vi "Get Validation Information From Module Connections.vi"(8 "error in":errorcluster, 10 "module connection information":T2[](array[typedef])) -> (0 "error out":errorcluster, 2 "validation information":T1)   [LabVIEW 2019, in "Routing and Faulting Scripting.lvlib"]
uses:
  Routing and Faulting Scripting.lvlib
  Types/Module Information.ctl
  Shared/Routing and Faulting Hardware API/Types/Possible Connections for Endpoint.ctl
  Validation Information.ctl
  Shared/Routing and Faulting Hardware API/Routing and Faulting Hardware API.lvlib
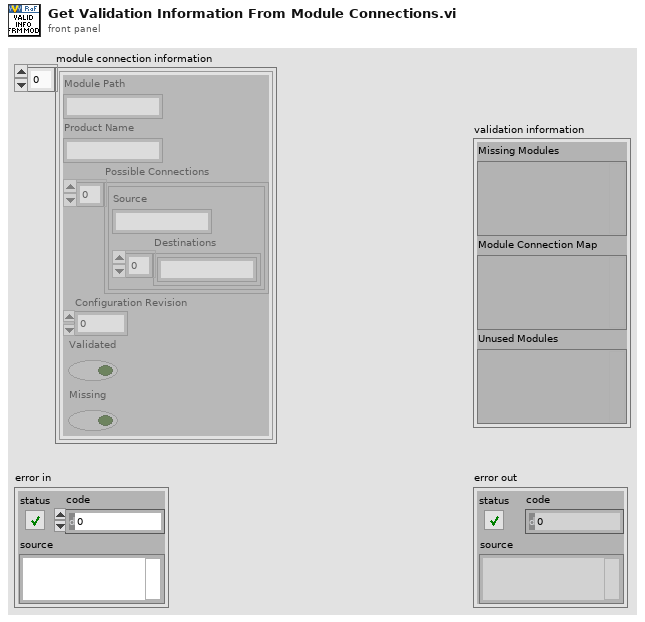
[diagram p1: front panel]
types:
  T1 = typedef "Routing and Faulting Scripting.lvlib/Validation Information.ctl" = cluster{"Missing Modules":variant, "Module Connection Map":variant, "Unused Modules":variant}
  T2 = typedef "Routing and Faulting Scripting.lvlib/Module Information.ctl" = cluster{"Module Path":string, "Product Name":string, "Possible Connections":T3[], "Configuration Revision":u32, "Validated":bool, "Missing":bool}
  T3 = typedef "Routing and Faulting Hardware API.lvlib/Possible Connections for Endpoint.ctl" = cluster{"Source":string, "Destinations":string[]}
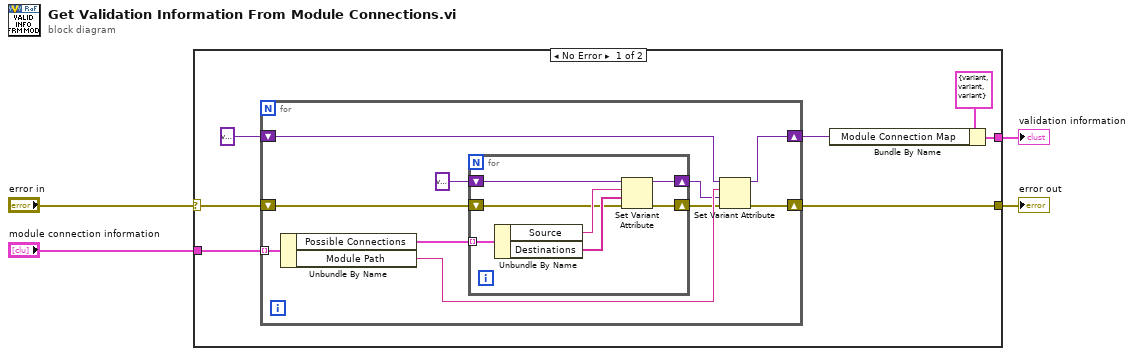
[diagram p0: block diagram]
diagram:
  n1 = case shown="No Error" "error in" {
    selector: "error in" -> [w5 w29]
    tunnel: "module connection information" -> [w8 _]
    tunnel: [w7 w29] -> w3
    tunnel: [w6 _] -> w2
    frame No Error {
      n2 = for {
        shift-right: [w12] -> w9
        shift-left: variant -> [w13]
        tunnel: w8 -> [w20] mode=indexing
        shift-right: [w14] -> w7
        shift-left: w5 -> [w16]
        n3 = Unbundle By Name(w20) -> ("Possible Connections"=w19:T3[], "Module Path"=w18:string)
        n4 = for {
          shift-right: [w24] -> w17
          shift-left: variant -> [w28]
          tunnel: w19 -> [w27] mode=indexing
          shift-right: [w22] -> w15
          shift-left: w16 -> [w23]
          n5 = Unbundle By Name(w27) -> ("Source"=w26:string, "Destinations"=w25:string[])
          n6 = Set Variant Attribute(Variant=w28, name=w26, value=w25, error in=w23) -> (Variant out=w24:variant, error out=w22:errorcluster)  [unwired: 1 out]
        }
        n7 = Set Variant Attribute(Variant=w13, name=w18, value=w17, error in=w15) -> (Variant out=w12:variant, error out=w14:errorcluster)  [unwired: 1 out]
      }
      n8 = Bundle By Name(cluster=T1 {"Missing Modules"=variant(cluster{"ID":string, "Path":string}[] []), "Module Connection Map"=variant, "Unused Modules"=variant(cluster{"ID":string, "Path":string}[] [])} ("Validation Information"), "Module Connection Map"=w9) -> (w6:T1)
    }
    frame Error {
    }
  }
  "error out" <- w3
  "validation information" <- w2
